vi "Configure Input Path.vi"(0 "VISA resource name":refnum<visa-resource-name>, 5 "Channel (4 = All)":enum16{"C1", "C2", "C3", "C4", "All"}(ring), 7 "Path (0 = A)":enum16{"A", "B"}(ring), 11 "error in (no error)":errorcluster) -> (4 "VISA resource name out":refnum<visa-resource-name>, 15 "error out":errorcluster)   [LabVIEW 2018, in "LeCroy Wave Series.lvlib"]
doc: "Configures the input path for a channel. This VI is only used for scopes that have tow rows of connectors for Probus vs Prolink inputs. The top row (\"A\") is for Prolink probes and for higher BW cable connections (typically using LP-SMA adapters.) The bottom row (B) is for lower bandwidth BNC connections and Probus-compatible probes.\n\nNote: This VI is only for use with certain model oscilloscopes."
uses:
  LeCroy Wave Series.lvlib
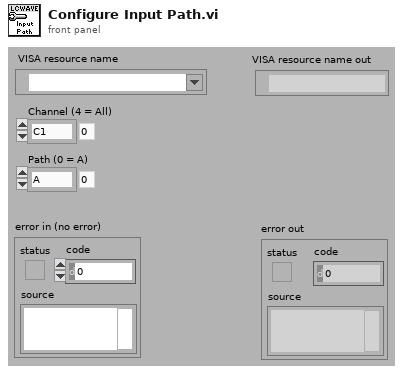
[diagram p1: front panel]
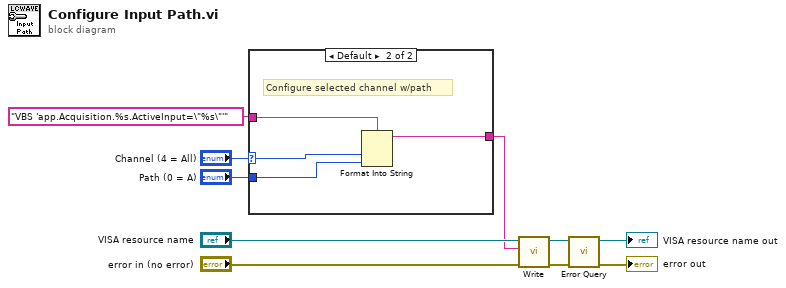
[diagram p0: block diagram]
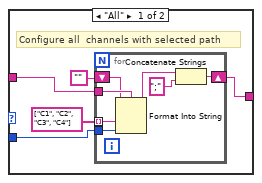
[diagram p2: hidden frame]
diagram:
  n1 = case shown="Default" "Channel (4 = All)" {
    selector: "Channel (4 = All)" -> [_ w26]
    tunnel: "VBS 'app.Acquisition.%s.ActiveInput=\"%s\"'" ("format string") -> [w12 w25]
    tunnel: [w15 w24] -> w2
    tunnel: "Path (0 = A)" -> [w13 w23]
    frame "All" {
      # "Configure all  channels with selected path"
      n2 = for {
        shift-right: [w22] -> w15
        shift-left: "" -> [w16]
        tunnel: string[] ["C1", "C2", "C3", "C4"] -> [w19] mode=indexing
        tunnel: w13 -> [w18]
        tunnel: w12 -> [w17]
        n3 = Format Into String(format string=w17, initial string=w16, w19, w18) -> (resulting string=w20:string)  [unwired: 1 in, 1 out]
        n4 = Concatenate Strings(w20, ";" ("string")) -> (w22:string)
      }
    }
    frame Default {
      # "Configure selected channel w/path"
      n5 = Format Into String(format string=w25, w26, w23) -> (resulting string=w24:string)  [unwired: 2 in, 1 out]
    }
  }
  n6 = call "Write.vi"("error in (no error)"="error in (no error)", "Write Buffer"=w2, "VISA resource name"="VISA resource name") -> ("error out"=w5:errorcluster, "VISA resource name out"=w6:refnum<visa-resource-name>)  [unwired: 7 in]
  n7 = call "Error Query.vi"("error in (no error)"=w5, "VISA resource name"=w6) -> ("error out"=→"error out":errorcluster, "VISA resource name out"=→"VISA resource name out":refnum<visa-resource-name>)  [unwired: 6 in, 2 out]
